vi "Random Number (Range) I64.vi"(10 "lower bound (-100)":i64=-100, 11 "upper bound (100)":i64=100) -> (3 "number":i64)   [LabVIEW 2020]
doc: "Generates a random value from a specified range. Wire data to the <B>upper bound</B> or <B>lower bound</B> input to determine the polymorphic instance to use or manually select the instance."
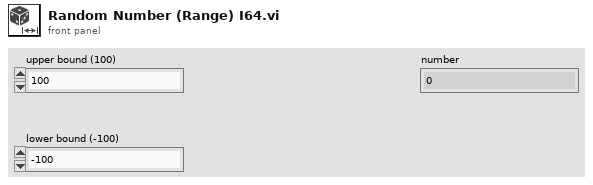
[diagram p1: front panel]
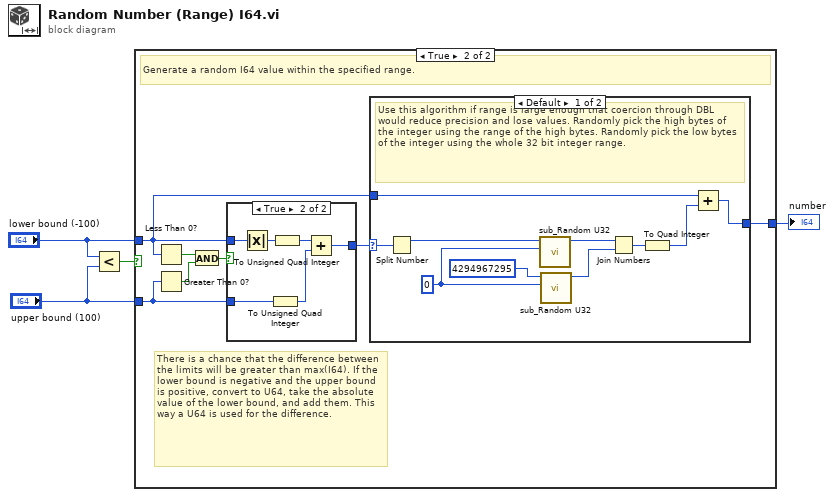
[diagram p0: block diagram]
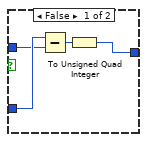
[diagram p3: hidden frame]
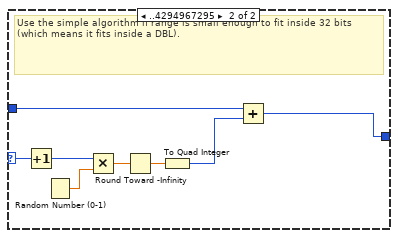
[diagram p4: hidden frame]
diagram:
  n1 = Less?(x="lower bound (-100)", y="upper bound (100)") -> (x < y?=w4:bool)
  n2 = case shown="True" w4 {
    tunnel: "lower bound (-100)" -> [w5 w10]
    tunnel: "upper bound (100)" -> [_ w9]
    tunnel: [w5 w11] -> w1
    frame False {
      # "If bounds are reversed, always return the lower bound."
    }
    frame True {
      # "There is a chance that the difference between the limits will be greater than max(I64). If the lower bound is negative and the upper bound is positive, convert to U64, take the absolute value of the lower bound, and add them. This way a U64 is used for the difference."
      # "Generate a random I64 value within the specified range."
      n3 = Less Than 0?(x=w10) -> (x < 0?=w8:bool)
      n4 = Greater Than 0?(x=w9) -> (x > 0?=w6:bool)
      n5 = And(x=w8, y=w6) -> (x .and. y?=w7:bool)
      n6 = case shown="True" w7 {
        tunnel: w9 -> [w16 w20]
        tunnel: [w13 w17] -> w12
        tunnel: w10 -> [w14 w22]
        frame False {
          n7 = Subtract(x=w16, y=w14) -> (x-y=w15:i64)
          n8 = To Unsigned Quad Integer(1:w15) -> (0:w13:u64)
        }
        frame True {
          n9 = Absolute Value(x=w22) -> (abs(x)=w21:i64)
          n10 = To Unsigned Quad Integer(1:w20) -> (0:w18:u64)
          n11 = To Unsigned Quad Integer(1:w21) -> (0:w19:u64)
          n12 = Add(x=w19, y=w18) -> (x+y=w17:u64)
        }
      }
      n13 = case shown="Default" w12 {
        selector: w12 -> [w32 w38]
        tunnel: w10 -> [w30 w40]
        tunnel: [w29 w39] -> w11
        frame Default {
          w27 = u32 0 ("lower bound")
          # "Use this algorithm if range is large enough that coercion through DBL would reduce precision and lose values. Randomly pick the high bytes of the integer using the range of the high bytes. Randomly pick the low bytes of the integer using the whole 32 bit integer range."
          n14 = Split Number(x=w32) -> (hi(x)=w28:u32)  [unwired: 1 out]
          n15 = call <vilib>:"sub_Random U32.vi"("lower bound"=w27, "upper bound"=w28) -> ("number"=w24:u32)  [unwired: 9 in]
          n16 = call <vilib>:"sub_Random U32.vi"("lower bound"=w27, "upper bound"=u32 4294967295) -> ("number"=w25:u32)  [unwired: 9 in]
          n17 = Join Numbers(hi=w24, lo=w25) -> ((hi.lo)=w31:u64)
          n18 = To Quad Integer(1:w31) -> (0:w23:i64)
          n19 = Add(x=w30, y=w23) -> (x+y=w29:i64)
        }
        frame ..4294967295 {
          # "Use the simple algorithm if range is small enough to fit inside 32 bits (which means it fits inside a DBL)."
          n20 = Increment(x=w38) -> (x+1=w37:u64)
          n21 = Random Number (0-1)() -> (number: 0 to 1=w36:dbl)
          n22 = Multiply(x=w37, y=w36) -> (x*y=w35:dbl)
          n23 = Round Toward -Infinity(1:w35) -> (0:w34:dbl)
          n24 = To Quad Integer(1:w34) -> (0:w33:i64)
          n25 = Add(x=w40, y=w33) -> (x+y=w39:i64)
        }
      }
    }
  }
  "number" <- w1
